vi "Write Key.vi"(8 "Error In":errorcluster, 10 "Key":string, 11 "Variable In":refnum<class "Keyable.lvclass">) -> (0 "Error Out":errorcluster, 3 "Variable Out":refnum<class "Keyable.lvclass">)   [LabVIEW 2018, in "Toolkit.lvlib" / "Tokens.lvlib" / "Keyable.lvclass"]
uses:
  API/Keyable.lvclass
  API/Keyable.lvclass/Keyable.ctl
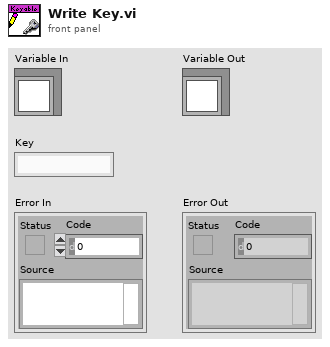
[diagram p1: front panel]
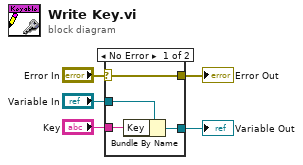
[diagram p0: block diagram]
diagram:
  n1 = case shown="No Error" "Error In" {
    selector: "Error In" -> [w9 w10]
    tunnel: [w9 w10] -> w4
    tunnel: [w7 w11] -> w2
    tunnel: "Variable In" -> [w8 w11]
    tunnel: "Key" -> [w6 _]
    frame No Error {
      n2 = Bundle By Name(cluster=w8, "Key"=w6) -> (w7:refnum<class "Keyable.lvclass">)
    }
    frame Error {
    }
  }
  "Error Out" <- w4
  "Variable Out" <- w2
